vi "ClearMessage.vi"(8 "error in (no error)":errorcluster) -> (0 "error out":errorcluster)   [LabVIEW 2013]
uses:
  030 - EVENTS/EnumFgvEventCommand.ctl
  030 - EVENTS/01 - ToHmiScheduler/ToHmiScheduler.ctl
  030 - EVENTS/01 - ToHmiScheduler/ToHmiSchedulerCommand.ctl
  030 - EVENTS/03 - ToMessageHandlerProcess/ToMessageHandlerEvent.ctl
  030 - EVENTS/03 - ToMessageHandlerProcess/enumMessageCriticity.ctl
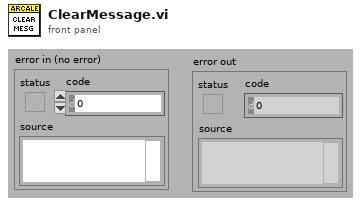
[diagram p1: front panel]
types:
  T1 = typedef "ToHmiSchedulerCommand.ctl" = enum16{"Load screen", "Lock screen", "Unlock screen", "Close enable", "Close disable", "Start automatic progress bar", "Stop automatic progress bar", "Set progress bar value (0..100)", "Load previous screen", "Close application", "View message", "Clear message", "Set Window State"}
  T2 = typedef "ToHmiScheduler.ctl" = cluster{"Command":T1, "Screen path":path, "Progress bar value":u8, "Screen Title":string, "To message handler event":T3, "Window_State":enum32{"Invalid", "Standard", "Closed", "Hidden", "Minimized", "Maximized"}}
  T3 = typedef "ToMessageHandlerEvent.ctl" = cluster{"date / time":timestamp, "Criticity":T4, "Emitter":string, "Message":string}
  T4 = typedef "enumMessageCriticity.ctl" = enum16{"No error", "Info", "Warning", "Error", "Fatal error"}
  T5 = typedef "EnumFgvEventCommand.ctl" = enum16{"Setup", "Cleanup", "Get"}
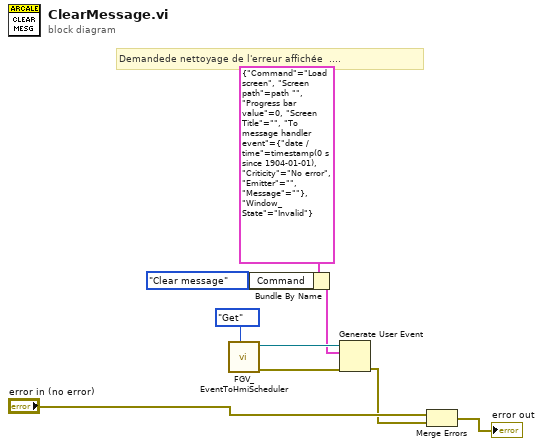
[diagram p0: block diagram]
diagram:
  # "Demandede nettoyage de l'erreur affichée  ...."
  n1 = call "FGV_EventToHmiScheduler.vi"("Command"=EnumFgvEventCommand."Get") -> ("error out"=w8:errorcluster, "ToHmiSchedulerEvent"=w7:refnum<user-event>)  [unwired: 9 in]
  n2 = Bundle By Name(cluster=T2 {"Command"=enum."Load screen", "Screen path"=path "", "Progress bar value"=0, "Screen Title"="", "To message handler event"={"date / time"=timestamp(0 s since 1904-01-01), "Criticity"=enum."No error", "Emitter"="", "Message"=""}, "Window_State"=enum."Invalid"} ("event data"), "Command"=ToHmiSchedulerCommand."Clear message") -> (w5:T2)
  n3 = Generate User Event(user event=w7, event data cluster=w5, error in=w8) -> (error out=w3:errorcluster)  [unwired: 1 in, 1 out]
  n4 = Merge Errors("error in (no error)", w3) -> (→"error out":errorcluster)
